vi "Configure Frequery and Level.vi"(4 "Current Level (1)":dbl=1.0 min=0.1 max=20.0 step=0.01, 6 "Voltage Level (1)":dbl=1.0 min=0.01 max=2.0 step=0.01, 7 "Level Mode":u16(ring) items=["Voltage", "Current"], 8 "error in (no error)":errorcluster, 9 "ALC (F: Disable)":bool, 10 "Frequery (1000)":dbl=1000.0 min=10.0 max=300000.0 step=0.01, 11 "VISA resource name":refnum<visa-resource-name>) -> (0 "error out":errorcluster, 3 "VISA resource name out":refnum<visa-resource-name>)   [LabVIEW 2021, in "LCR Meter.lvlib"]
doc: "Configure the Frequery and Level."
uses:
  LCR Meter.lvlib
panel:
  # "Hz"
  # "V"
  # "mA"
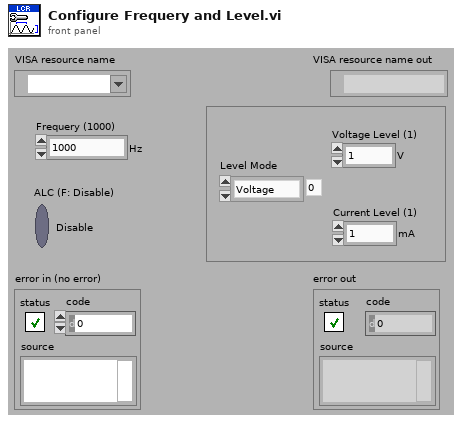
[diagram p1: front panel]
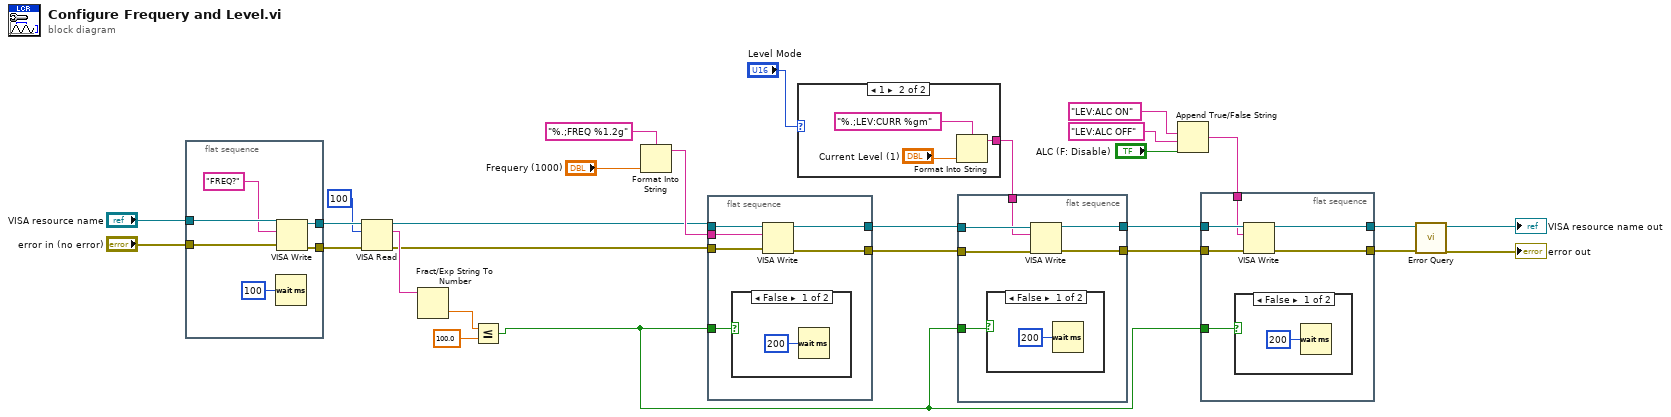
[diagram p0: block diagram]
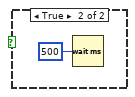
[diagram p2: hidden frame]
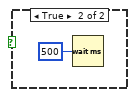
[diagram p3: hidden frame]
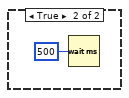
[diagram p4: hidden frame]
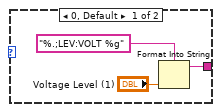
[diagram p5: hidden frame]
diagram:
  n1 = flat-sequence {
    tunnel: "VISA resource name" -> [w34]
    tunnel: "error in (no error)" -> [w33]
    tunnel: [w30] -> w9
    tunnel: [w29] -> w8
    frame #0 {
      n2 = Wait (ms)(milliseconds to wait=u32 100) -> ()  [unwired: 1 out]
      n3 = VISA Write(VISA resource name=w34, write buffer="FREQ?", error in (no error)=w33) -> (VISA resource name out=w30:refnum<visa-resource-name>, error out=w29:errorcluster)  [unwired: 1 out]
    }
  }
  n4 = VISA Read(VISA resource name=w9, byte count=u32 100, error in (no error)=w8) -> (VISA resource name out=w6:refnum<visa-resource-name>, read buffer=w7:string, error out=w5:errorcluster)  [unwired: 1 out]
  n5 = Fract/Exp String To Number(string=w7) -> (number=w3:dbl)  [unwired: 3 in, 1 out]
  n6 = Less Or Equal?(x=w3, y=100.0) -> (x <= y?=w1:bool)
  n7 = Format Into String(format string="%.;FREQ %1.2g", "Frequery (1000)") -> (resulting string=w22:string)  [unwired: 2 in, 1 out]
  n8 = flat-sequence {
    tunnel: w22 -> [w40]
    tunnel: w6 -> [w39]
    tunnel: w5 -> [w38]
    tunnel: [w37] -> w15
    tunnel: [w36] -> w14
    tunnel: w1 -> [w35]
    frame #0 {
      n9 = case shown="False" w35 {
        frame False {
          n10 = Wait (ms)(milliseconds to wait=u32 200) -> ()  [unwired: 1 out]
        }
        frame True {
          n11 = Wait (ms)(milliseconds to wait=u32 500) -> ()  [unwired: 1 out]
        }
      }
      n12 = VISA Write(VISA resource name=w39, write buffer=w40, error in (no error)=w38) -> (VISA resource name out=w37:refnum<visa-resource-name>, error out=w36:errorcluster)  [unwired: 1 out]
    }
  }
  n13 = case shown="1" "Level Mode" {
    tunnel: [w45 w48] -> w21
    frame 0, Default {
      n14 = Format Into String(format string="%.;LEV:VOLT %g", "Voltage Level (1)") -> (resulting string=w45:string)  [unwired: 2 in, 1 out]
    }
    frame 1 {
      n15 = Format Into String(format string="%.;LEV:CURR %gm", "Current Level (1)") -> (resulting string=w48:string)  [unwired: 2 in, 1 out]
    }
  }
  n16 = flat-sequence {
    tunnel: w15 -> [w54]
    tunnel: w14 -> [w53]
    tunnel: w21 -> [w52]
    tunnel: [w51] -> w13
    tunnel: [w50] -> w12
    tunnel: w1 -> [w49]
    frame #0 {
      n17 = case shown="False" w49 {
        frame False {
          n18 = Wait (ms)(milliseconds to wait=u32 200) -> ()  [unwired: 1 out]
        }
        frame True {
          n19 = Wait (ms)(milliseconds to wait=u32 500) -> ()  [unwired: 1 out]
        }
      }
      n20 = VISA Write(VISA resource name=w54, write buffer=w52, error in (no error)=w53) -> (VISA resource name out=w51:refnum<visa-resource-name>, error out=w50:errorcluster)  [unwired: 1 out]
    }
  }
  n21 = Append True/False String(1:"ALC (F: Disable)", 2:"LEV:ALC OFF", 3:"LEV:ALC ON") -> (0:w19:string)  [unwired: 1 in]
  n22 = flat-sequence {
    tunnel: w13 -> [w62]
    tunnel: w12 -> [w61]
    tunnel: [w60] -> w18
    tunnel: [w59] -> w17
    tunnel: w19 -> [w58]
    tunnel: w1 -> [w57]
    frame #0 {
      n23 = case shown="False" w57 {
        frame False {
          n24 = Wait (ms)(milliseconds to wait=u32 200) -> ()  [unwired: 1 out]
        }
        frame True {
          n25 = Wait (ms)(milliseconds to wait=u32 500) -> ()  [unwired: 1 out]
        }
      }
      n26 = VISA Write(VISA resource name=w62, write buffer=w58, error in (no error)=w61) -> (VISA resource name out=w60:refnum<visa-resource-name>, error out=w59:errorcluster)  [unwired: 1 out]
    }
  }
  n27 = call "Error Query.vi"("error in (no error)"=w17, "VISA resource name"=w18) -> ("error out"=→"error out":errorcluster, "VISA resource name out"=→"VISA resource name out":refnum<visa-resource-name>)  [unwired: 6 in, 2 out]
